vi "TDS_SaveConfigurationToFile.vi"(8 "error in":errorcluster, 11 "VI Server ClusterDUP":T1) -> (0 "error out":errorcluster)   [LabVIEW 2020]
uses:
  LabVIEW 2020 Toolkits/VI Server Toolkit/VI Server_TypeDefs/VI Server_RefsCluster.ctl
  LabVIEW 2020 Toolkits/VI Server Toolkit/VI Server Libraries/VI Server Controls.llb/VI Server_GetSet Controls From String Format_Options.ctl
  LabVIEW 2020 Toolkits/VI Server Toolkit/VI Server Libraries/VI Server_GetControl.llb/VI Server_PATH_Get.vi
  LabVIEW 2020 Toolkits/VI Server Toolkit/VI Server Libraries/VI Server_GetControl.llb/VI Server_STR_Get.vi
  <vilib>/Utility/config.llb/Write Key (String).vi
  LabVIEW 2020 Toolkits/VI Server Toolkit/VI Server Toolkit LV2013.lvlib
  <vilib>/Utility/config.llb/NI_LVConfig.lvlib
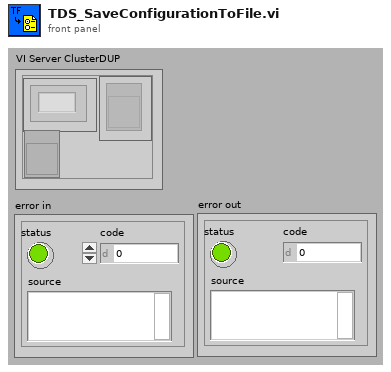
[diagram p1: front panel]
types:
  T1 = typedef "VI Server_RefsCluster.ctl" = cluster{"Labels":string[], "Refs":refnum<vi>[], "VI Ref":refnum<vi>}
  T2 = typedef "VI Server Toolkit LV2013.lvlib/VI Server_GetSet Controls From String Format_Options.ctl" = enum16{"", "If Ring Get Selection", "If Ring Set by Selection"}
  T3 = typedef "NI_LVConfig.lvlib/Config Data RefNum.ctl" = refnum<k1>
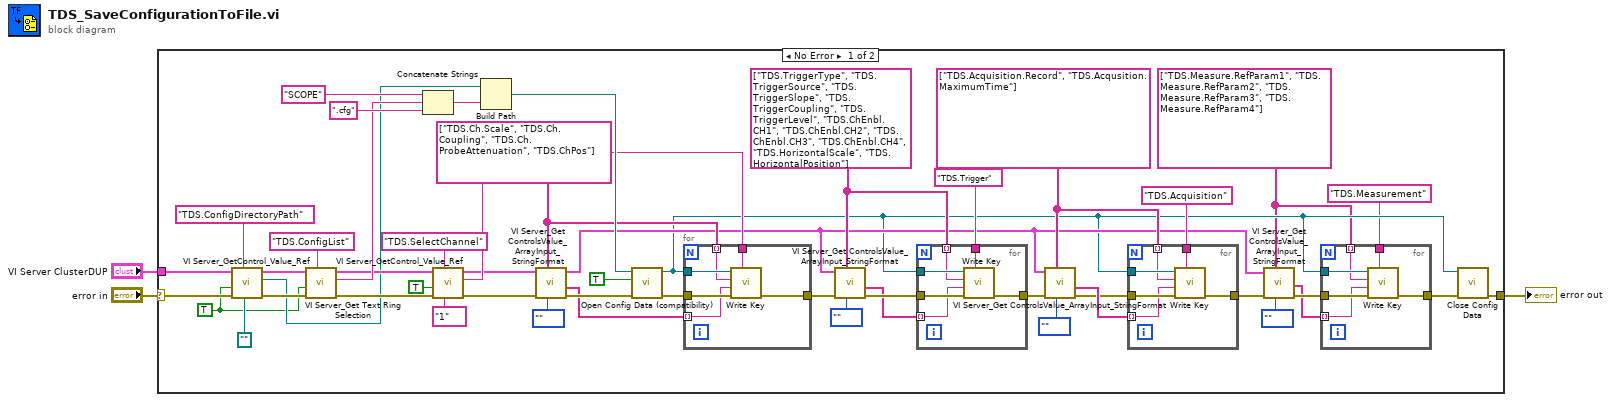
[diagram p0: block diagram]
diagram:
  n1 = case shown="No Error" "error in" {
    selector: "error in" -> [w24 w78]
    tunnel: "VI Server ClusterDUP" -> [w22 _]
    tunnel: [w40 w78] -> w2
    frame No Error {
      w6 = TRUE ("SingleInstance")
      w12 = string[] ["TDS.Measure.RefParam1", "TDS.Measure.RefParam2", "TDS.Measure.RefParam3", "TDS.Measure.RefParam4"]
      w25 = string[] ["TDS.Acquisition.Record", "TDS.Acqusition.MaximumTime"]
      w35 = string[] ["TDS.Ch.Scale", "TDS.Ch.Coupling", "TDS.Ch.ProbeAttenuation", "TDS.ChPos"]
      w32 = string[] ["TDS.TriggerType", "TDS.TriggerSource", "TDS.TriggerSlope", "TDS.TriggerCoupling", "TDS.TriggerLevel", "TDS.ChEnbl.CH1", "TDS.ChEnbl.CH2", "TDS.ChEnbl.CH3", "TDS.ChEnbl.CH4", "TDS.HorizontalScale", "TDS.HorizontalPosition"]
      n2 = call-poly "VI Server_GetControl_Value_Ref.vi"("DataType"=path "", "Control.Label"="TDS.ConfigDirectoryPath" ("Label"), "error in"=w24, "SingleInstance"=w6, "VI Server.RefsCluster"=w22) -> ("error out"=w23:errorcluster, "Value"=w18:path, "VI Server.RefsCluster.DUP"=w21:T1)  [unwired: 3 in, 1 out]
      n3 = call "VI Server_Get Text Ring Selection.vi"("Label"="TDS.ConfigList", "error in"=w23, "Single Instance (T)"=w6, "VI Server Cluster"=w21) -> ("error out"=w47:errorcluster, "Selection"=w51:string, "VI Server Custer.DUP"=w48:T1)  [unwired: 2 in, 3 out]
      n4 = Concatenate Strings("SCOPE" ("regular expression"), w51, ".cfg" ("string")) -> (w49:string)
      n5 = call-poly "VI Server_GetControl_Value_Ref.vi"("DataType"="1" ("Default Value"), "Control.Label"="TDS.SelectChannel" ("Label"), "error in"=w47, "SingleInstance"=TRUE, "VI Server.RefsCluster"=w48) -> ("error out"=w38:errorcluster, "Value"=w41:string, "VI Server.RefsCluster.DUP"=w37:T1)  [unwired: 3 in, 1 out]
      n6 = Build Path(base path=w18, name or relative path=w49) -> (appended path=w46:path)
      n7 = call "VI Server_Get ControlsValue_ArrayInput_StringFormat.vi"("Options"=VI_Server_GetSet_Controls_From_String_Format_Options."", "Labels.Array"=w35, "error in (no error)"=w38, "VI Server Cluster"=w37) -> ("error out"=w36:errorcluster, "Values.Array.STR"=w34:string[], "VI Server Cluster.DUP"=w16:T1)  [unwired: 3 in, 2 out]
      n8 = call <vilib>:"Open Config Data (compatibility).vi"("error in (no error)"=w36, "create file if necessary (T)"=TRUE ("create file if necessary? (T)"), "configuration file path"=w46) -> ("error out"=w42:errorcluster, "refnum"=w13:T3)  [unwired: 6 in, 1 out]
      n9 = for {
        tunnel: w42 -> [w77]
        tunnel: w13 -> [w76]
        tunnel: [w75] -> w33
        tunnel: w41 -> [w74]
        tunnel: w34 -> [w73] mode=indexing
        tunnel: w35 -> [w72] mode=indexing
        n10 = call-poly <vilib>:"Write Key.vi"("section"=w74, "error in (no error)"=w77, "value"=w73, "key"=w72, "refnum"=w76) -> ("error out"=w75:errorcluster)  [unwired: 4 in, 2 out]
      }
      n11 = call "VI Server_Get ControlsValue_ArrayInput_StringFormat.vi"("Options"=VI_Server_GetSet_Controls_From_String_Format_Options."", "Labels.Array"=w32, "error in (no error)"=w33, "VI Server Cluster"=w16) -> ("error out"=w31:errorcluster, "Values.Array.STR"=w30:string[])  [unwired: 3 in, 3 out]
      n12 = for {
        tunnel: w31 -> [w71]
        tunnel: w13 -> [w70]
        tunnel: [w69] -> w26
        tunnel: "TDS.Trigger" -> [w68]
        tunnel: w30 -> [w66] mode=indexing
        tunnel: w32 -> [w67] mode=indexing
        n13 = call-poly <vilib>:"Write Key.vi"("section"=w68, "error in (no error)"=w71, "value"=w66, "key"=w67, "refnum"=w70) -> ("error out"=w69:errorcluster)  [unwired: 4 in, 2 out]
      }
      n14 = call "VI Server_Get ControlsValue_ArrayInput_StringFormat.vi"("Options"=VI_Server_GetSet_Controls_From_String_Format_Options."", "Labels.Array"=w25, "error in (no error)"=w26, "VI Server Cluster"=w16) -> ("error out"=w28:errorcluster, "Values.Array.STR"=w29:string[])  [unwired: 3 in, 3 out]
      n15 = for {
        tunnel: w28 -> [w65]
        tunnel: w13 -> [w64]
        tunnel: [w63] -> w17
        tunnel: "TDS.Acquisition" -> [w62]
        tunnel: w29 -> [w60] mode=indexing
        tunnel: w25 -> [w61] mode=indexing
        n16 = call-poly <vilib>:"Write Key.vi"("section"=w62, "error in (no error)"=w65, "value"=w60, "key"=w61, "refnum"=w64) -> ("error out"=w63:errorcluster)  [unwired: 4 in, 2 out]
      }
      n17 = call "VI Server_Get ControlsValue_ArrayInput_StringFormat.vi"("Options"=VI_Server_GetSet_Controls_From_String_Format_Options."", "Labels.Array"=w12, "error in (no error)"=w17, "VI Server Cluster"=w16) -> ("error out"=w15:errorcluster, "Values.Array.STR"=w11:string[])  [unwired: 3 in, 3 out]
      n18 = for {
        tunnel: w15 -> [w59]
        tunnel: w13 -> [w58]
        tunnel: [w57] -> w14
        tunnel: "TDS.Measurement" -> [w56]
        tunnel: w11 -> [w54] mode=indexing
        tunnel: w12 -> [w55] mode=indexing
        n19 = call-poly <vilib>:"Write Key.vi"("section"=w56, "error in (no error)"=w59, "value"=w54, "key"=w55, "refnum"=w58) -> ("error out"=w57:errorcluster)  [unwired: 4 in, 2 out]
      }
      n20 = call <vilib>:"Close Config Data.vi"("error in (no error)"=w14, "refnum"=w13) -> ("error out"=w40:errorcluster)  [unwired: 8 in, 1 out]
    }
    frame Error {
    }
  }
  "error out" <- w2
